vi "update_weight.vi"(8 "delta_value":dbl) -> ()   [LabVIEW 2014]
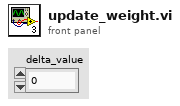
[diagram p1: front panel]
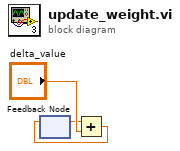
[diagram p0: block diagram]
diagram:
  n1 = feedback #1() -> (w1:dbl)  [unwired: 1 in]
  n2 = Add(x=w1, y="delta_value") -> (x+y=w2:dbl)
  n3 = feedback-in #1(w2) -> ()
